vi "Remap Demo.vi"() -> ()   [LabVIEW 2018]
uses:
  <vilib>/vision/NI_Vision_Development_Module.lvlib
  RemapDemo/LV_RemapOpenCV/x64/Release/LVRemapOpenCV.dll
panel:
  out "Image dst":T1(plugin-control)
  out "Pattern":T1(plugin-control)
  out "Image src":T1(plugin-control)
  out "Grid":T1(plugin-control)
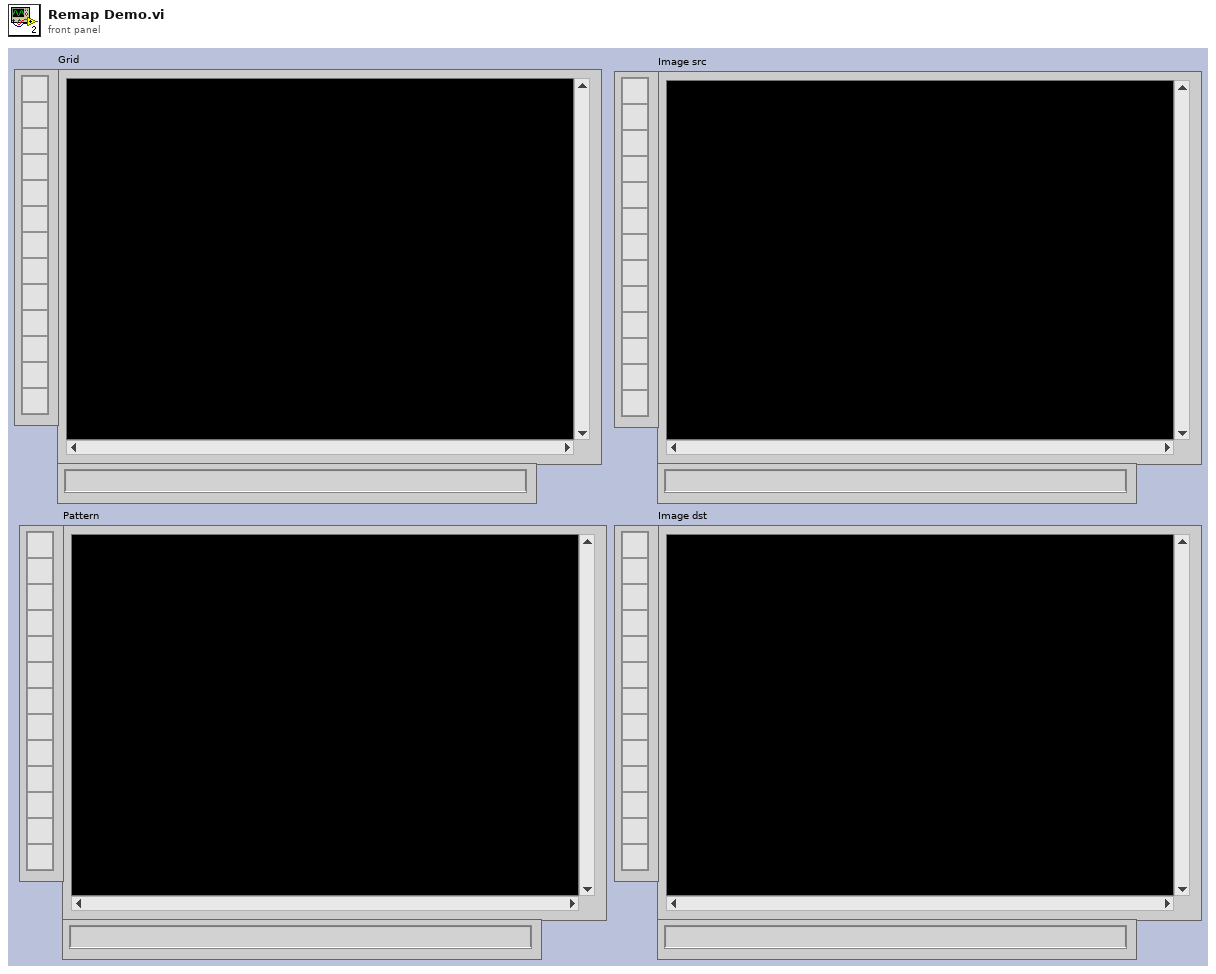
[diagram p1: front panel]
types:
  T1 = typedef "IMAQ Image.ctl" = refnum<image>
  T2 = typedef "Image Unit" = enum32{"Undefined", "Angström", "Micrometer", "Millimeter", "Centimeter", "Meter", "Kilometer", "Microinch", "Inch", "Feet", "Nautical miles", "Standard miles", "Steps"}
  T3 = typedef "Particle Parameters" = i32
  T4 = cluster{"Measurement Parameter":T3, "Range Lower Value":dbl, "Range Upper Value":dbl, "Range":bool, "Measurement Type":bool}[]
  T5 = typedef "Calibration Reference Points.ctl" = cluster{"Pixel Coordinates":cluster{"X":dbl, "Y":dbl}[], "Real World Coordinates":cluster{"X":dbl, "Y":dbl}[], "Unit":T2, "Image Size":cluster{"X":u32, "Y":u32}}
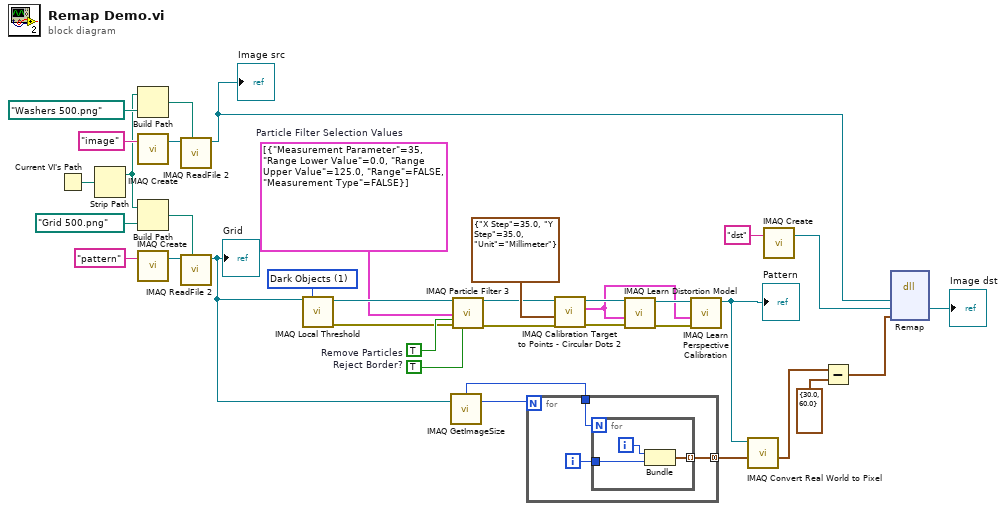
[diagram p0: block diagram]
diagram:
  w18 = T4 [{"Measurement Parameter"=35, "Range Lower Value"=0.0, "Range Upper Value"=125.0, "Range"=FALSE, "Measurement Type"=FALSE}]  # Particle Filter Selection Values
  w21 = TRUE  # Remove Particles
  w20 = TRUE  # Reject Border?
  w26 = u32 1 items=["Bright Objects", "Dark Objects"] ("Look For (Bright Objects)")
  n1 = Current VI's Path() -> (path=w36:path)
  n2 = Strip Path(path=w36) -> (stripped path=w27:path)  [unwired: 1 out]
  n3 = Build Path(base path=w27, name or relative path=path "Washers 500.png") -> (appended path=w30:path)
  n4 = call "IMAQ Create"("Image Name"="image") -> ("New Image"=w31:T1)  [unwired: 4 in, 1 out]
  n5 = Build Path(base path=w27, name or relative path=path "Grid 500.png") -> (appended path=w33:path)
  n6 = call "IMAQ Create"("Image Name"="pattern") -> ("New Image"=w32:T1)  [unwired: 4 in, 1 out]
  n7 = call "IMAQ ReadFile 2"("File Path"=w30, "Image"=w31) -> ("Image Out"=w5:T1)  [unwired: 5 in, 4 out]
  "Image src" <- w5
  n8 = call "IMAQ ReadFile 2"("File Path"=w33, "Image"=w32) -> ("Image Out"=w2:T1)  [unwired: 5 in, 4 out]
  "Grid" <- w2
  n9 = call "IMAQ Local Threshold"("Image Src"=w2, "Look For (Bright Objects)"=w26) -> ("Image Dst Out"=w19:T1, "error out"=w17:errorcluster)  [unwired: 7 in, 5 out]
  n10 = call "IMAQ GetImageSize"("Image"=w2) -> ("Y Resolution"=w3:i32, "X Resolution"=w4:i32)  [unwired: 3 in, 1 out]
  n11 = call "IMAQ Particle Filter 3"("Image Src"=w19, "Selection Values"=w18, "Keep/Remove Particles (F)"=w21, "error in (no error)"=w17, "Reject Border? (F)"=w20) -> ("Image Dst Out"=w13:T1, "error out"=w16:errorcluster)  [unwired: 4 in, 5 out]
  n12 = for {
    N: w3 -> [_]
    tunnel: [w38] -> w9 mode=concatenating
    tunnel: w4 -> [w37]
    i -> [w39]
    n13 = for {
      N: w37 -> [_]
      tunnel: w39 -> [w41]
      tunnel: [w40] -> w38 mode=indexing
      i -> [w42]
      n14 = Bundle(w42, w41) -> (w40:cluster{i32, i32})  [unwired: 1 in]
    }
  }
  n15 = call "IMAQ Calibration Target to Points - Circular Dots 2"("error in (no error)"=w16, "Grid Descriptor"=cluster{"X Step":sgl, "Y Step":sgl, "Unit":T2} {"X Step"=35.0, "Y Step"=35.0, "Unit"=enum."Millimeter"}, "Target Image"=w13) -> ("error out"=w15:errorcluster, "Reference Points"=w23:T5, "Target Image (dup)"=w25:T1)  [unwired: 6 in]
  n16 = call "IMAQ Learn Distortion Model"("error in (no error)"=w15, "Reference Points"=w23, "Calibration Template Image"=w25) -> ("error out"=w14:errorcluster, "Calibration Template Image Out"=w24:T1)  [unwired: 3 in, 4 out]
  n17 = call "IMAQ Learn Perspective Calibration"("error in (no error)"=w14, "Reference Points"=w23, "Calibration Template Image"=w24) -> ("Calibration Template Image Out"=w1:T1)  [unwired: 1 in, 7 out]
  "Pattern" <- w1
  n18 = call "IMAQ Convert Real World to Pixel"("Array of Real World Coordinates"=w9, "Calibrated Image"=w1) -> ("Array of Pixel Coordinates"=w8:cluster{"X":sgl, "Y":sgl}[])  [unwired: 4 in, 5 out]
  n19 = call "IMAQ Create"("Image Name"="dst") -> ("New Image"=w11:T1)  [unwired: 4 in, 1 out]
  n20 = Subtract(x=w8, y=cluster{"X":sgl, "Y":sgl} {"X"=30.0, "Y"=60.0}) -> (x-y=w7:cluster{"X":sgl, "Y":sgl}[])
  n21 = dll-call lib="C:/Users/108003658/OneDrive - Baker Hughes/Desktop/RemapDemo/LV_RemapOpenCV/x64/Release/LVRemapOpenCV.dll" fn="Remap"("arg1"=w5, "arg2"=w11, "XYmap"=w7) -> ("arg2"=→"Image dst":T1)  [unwired: 6 in, 2 out]
